vi "ReadData.vi"(8 "error in (no error)":errorcluster, 11 "Protocol In":refnum<class "Protocol.lvclass">) -> (0 "error out":errorcluster, 1 "read buffer":string, 3 "Protocol Out":refnum<class "Protocol.lvclass">)   [LabVIEW 2019, in "Protocol.lvclass"]
uses:
  Protocol.lvclass
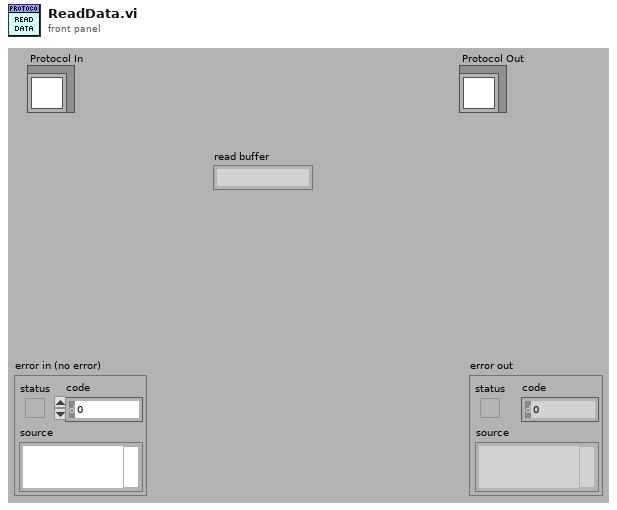
[diagram p1: front panel]
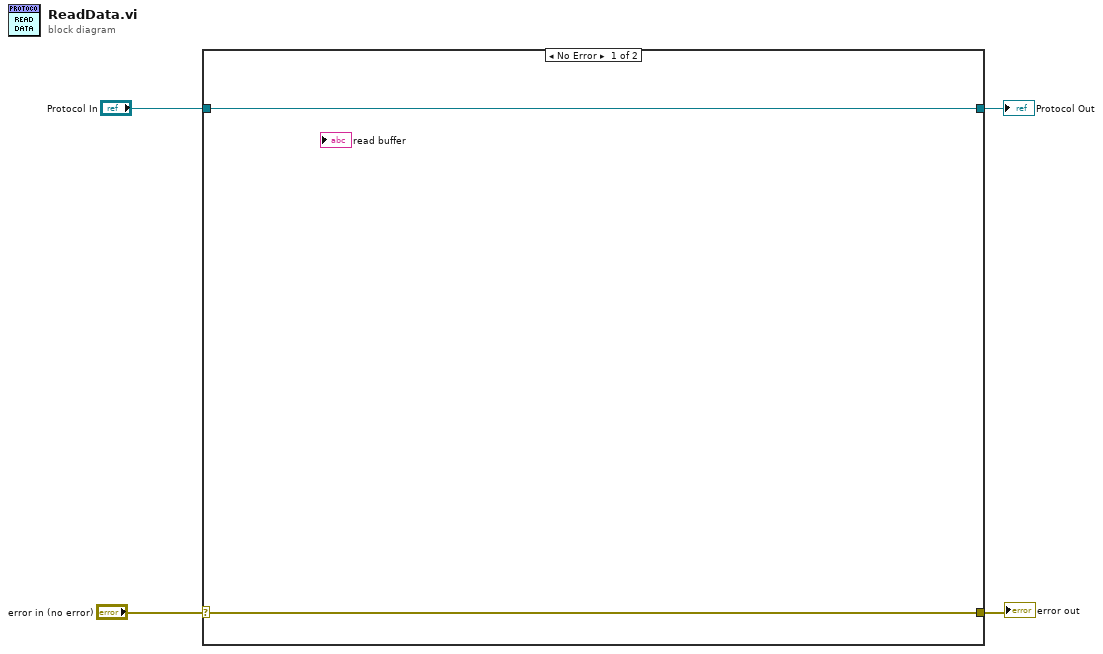
[diagram p0: block diagram]
diagram:
  n1 = case shown="No Error" "error in (no error)" {
    selector: "error in (no error)" -> [w6 w8]
    tunnel: [w6 w8] -> w3
    tunnel: [w5 w7] -> w1
    tunnel: "Protocol In" -> [w5 w7]
    frame No Error {
    }
    frame Error {
    }
  }
  "error out" <- w3
  "Protocol Out" <- w1
